vi "Configure Data Buffer.vi"(7 "Enable Data Buffer (T: Enable)":bool=TRUE, 8 "error in (no error)":errorcluster, 10 "Trace Data Source (0: Raw Data)":u16(ring) items=["Raw Data", "Math Data", "Limit Data"], 11 "VISA resource name":refnum<visa-resource-name>) -> (0 "error out":errorcluster, 3 "VISA resource name out":refnum<visa-resource-name>)   [LabVIEW 2012, in "Keithley 24XX.lvlib"]
doc: "Configures data buffer."
uses:
  <instrlib>/Keithley 24XX/Keithley 24XX.lvlib
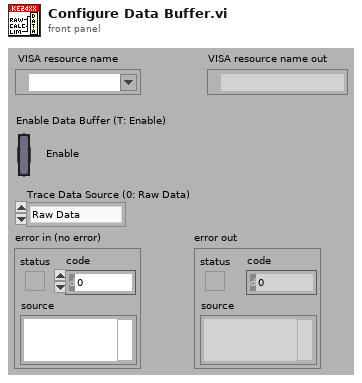
[diagram p1: front panel]
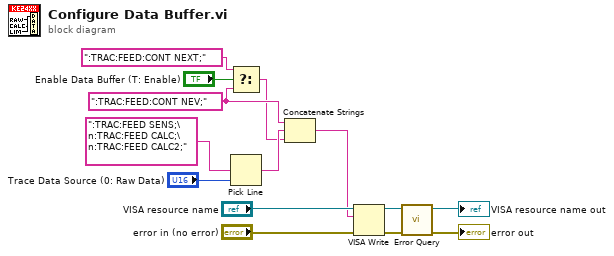
[diagram p0: block diagram]
diagram:
  w8 = ":TRAC:FEED:CONT NEV;"
  n1 = Select(t=":TRAC:FEED:CONT NEXT;", s="Enable Data Buffer (T: Enable)", f=w8) -> (s? t:f=w6:string)
  n2 = Pick Line(multi-line string=":TRAC:FEED SENS;\n:TRAC:FEED CALC;\n:TRAC:FEED CALC2;", line index="Trace Data Source (0: Raw Data)") -> (output string=w7:string)  [unwired: 1 in]
  n3 = Concatenate Strings(w8, w7, w6) -> (w5:string)
  n4 = VISA Write(VISA resource name="VISA resource name", write buffer=w5, error in (no error)="error in (no error)") -> (VISA resource name out=w4:refnum<visa-resource-name>, error out=w3:errorcluster)  [unwired: 1 out]
  n5 = call <instrlib>:"Error Query.vi"("error in (no error)"=w3, "VISA resource name"=w4) -> ("error out"=→"error out":errorcluster, "VISA resource name out"=→"VISA resource name out":refnum<visa-resource-name>)  [unwired: 6 in, 2 out]
